vi "Configure Measurement (Burst Power).vi"(0 "VISA resource name":refnum<visa-resource-name>, 1 "Auto Burst Width Mode (T: Enable)":bool=TRUE, 2 "Manual Burst Width (0.0002556 s)":dbl=0.0002556, 5 "Threshold Type (0: Relative)":i32(ring) items=["Relative", "Absolute"], 7 "Threshold Level (-30 dB)":dbl=-30.0, 9 "Measurement Method (0: Above Threshold)":i32(ring) items=["Above Threshold Level", "Measured Burst Width"], 11 "error in (no error)":errorcluster, 12 "Bandwidth Filter Type (0: Gaussian)":i32(ring) items=["Gaussian", "Flattop"]) -> (4 "VISA resource name out":refnum<visa-resource-name>, 15 "error out":errorcluster)   [LabVIEW 2014, in "Agilent MXA Series.lvlib"]
doc: "Sets the Burst Power measurement parameters."
uses:
  Agilent MXA Series.lvlib
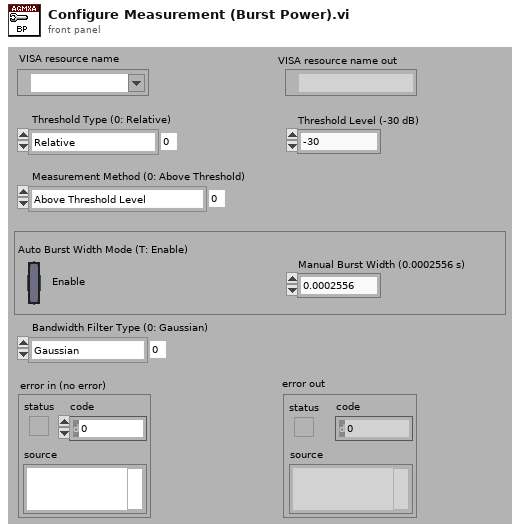
[diagram p1: front panel]
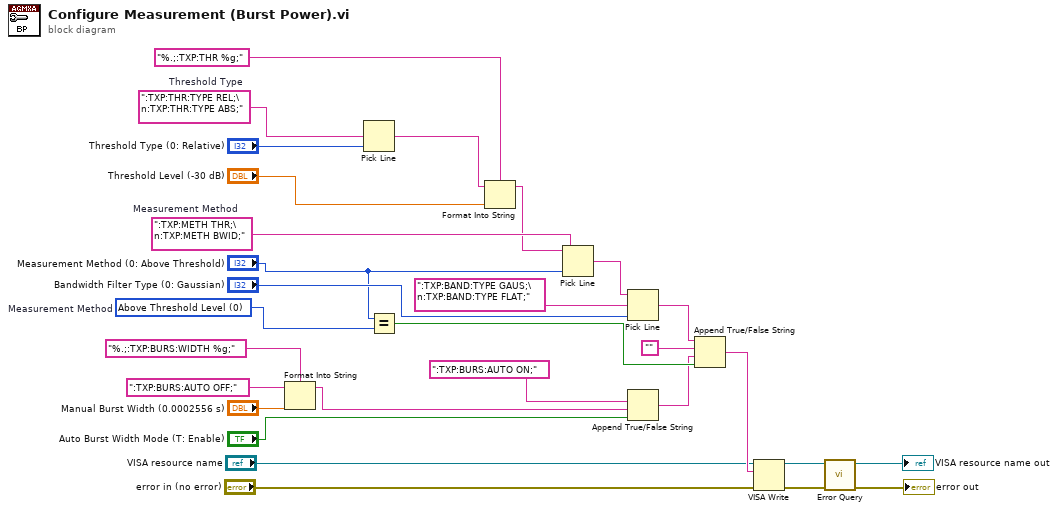
[diagram p0: block diagram]
diagram:
  w1 = 0 items=["Above Threshold Level", "Measured Burst Width"]  # Measurement Method
  w24 = ":TXP:METH THR;\n:TXP:METH BWID;"  # Measurement Method
  w28 = ":TXP:THR:TYPE REL;\n:TXP:THR:TYPE ABS;"  # Threshold Type
  n1 = Format Into String(format string="%.;:TXP:BURS:WIDTH %g;", initial string=":TXP:BURS:AUTO OFF;", "Manual Burst Width (0.0002556 s)") -> (resulting string=w15:string)  [unwired: 1 in, 1 out]
  n2 = Pick Line(multi-line string=w28, line index="Threshold Type (0: Relative)") -> (output string=w25:string)  [unwired: 1 in]
  n3 = Equal?(x="Measurement Method (0: Above Threshold)", y=w1) -> (x = y?=w13:bool)
  n4 = Format Into String(format string="%.;:TXP:THR %g;", initial string=w25, "Threshold Level (-30 dB)") -> (resulting string=w23:string)  [unwired: 1 in, 1 out]
  n5 = Pick Line(string ("")=w23, multi-line string=w24, line index="Measurement Method (0: Above Threshold)") -> (output string=w21:string)
  n6 = Pick Line(string ("")=w21, multi-line string=":TXP:BAND:TYPE GAUS;\n:TXP:BAND:TYPE FLAT;", line index="Bandwidth Filter Type (0: Gaussian)") -> (output string=w12:string)
  n7 = Append True/False String(1:"Auto Burst Width Mode (T: Enable)", 2:w15, 3:":TXP:BURS:AUTO ON;" ("true string")) -> (0:w10:string)  [unwired: 1 in]
  n8 = Append True/False String(1:w13, 2:w10, 3:"" ("true string"), 4:w12) -> (0:w9:string)
  n9 = VISA Write(VISA resource name="VISA resource name", write buffer=w9, error in (no error)="error in (no error)") -> (VISA resource name out=w5:refnum<visa-resource-name>, error out=w6:errorcluster)  [unwired: 1 out]
  n10 = call "Error Query.vi"("error in (no error)"=w6, "VISA resource name"=w5) -> ("error out"=→"error out":errorcluster, "VISA resource name out"=→"VISA resource name out":refnum<visa-resource-name>)  [unwired: 6 in, 2 out]
